vi "Get Output Values.vi"(8 "error in (no error)":errorcluster, 10 "Number of points":i32, 11 "Spectrum Recorder in":refnum<class "Spectrum Recorder.lvclass">) -> (0 "error out":errorcluster, 2 "Output values":dbl[](array[numeric]), 3 "Spectrum Recorder out":refnum<class "Spectrum Recorder.lvclass">)   [LabVIEW 2016, in "Spectrum Recorder.lvclass"]
uses:
  Spectrum Recorder.lvclass
  D:/github/Measure_core/Instrument Actor/Instrument Actor.lvclass
  Spectrum Recorder.lvclass/Spectrum Recorder.ctl
  Read Spectrum Recorder Configuration.vi
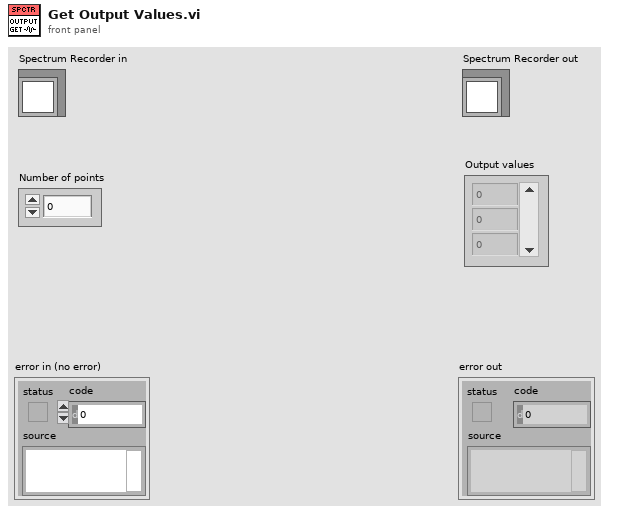
[diagram p1: front panel]
types:
  T1 = typedef "Spectrum Recorder Configuration.ctl" = cluster{"Start":dbl, "End":dbl, "Duration":dbl, "Filter time constant":dbl, "Repeat (-1: forever)":i32, "Update rate":dbl, "Data storage folder":path}
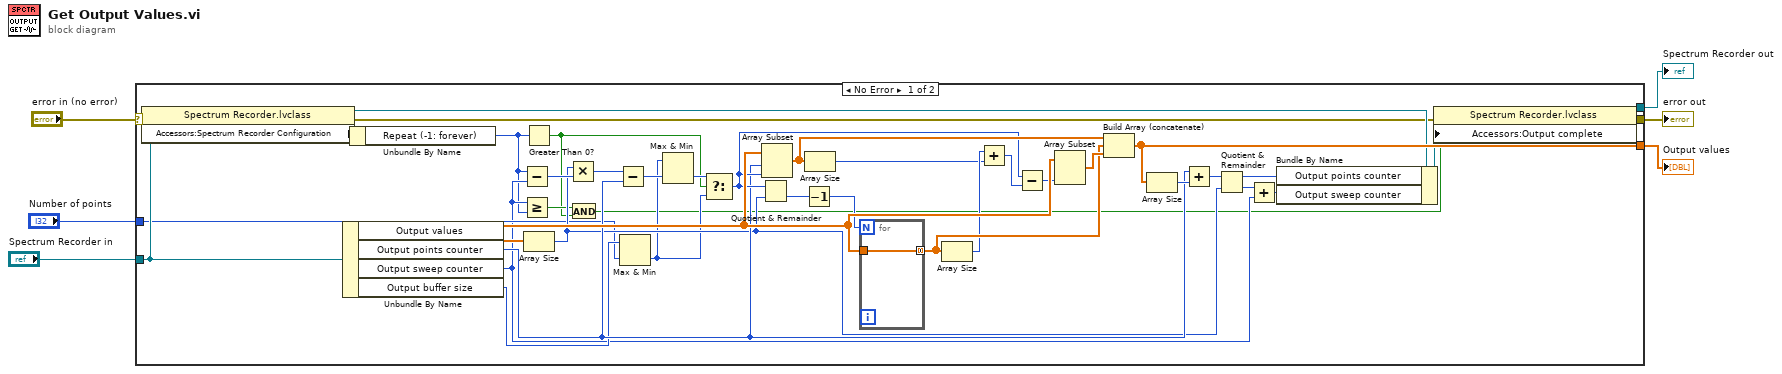
[diagram p0: block diagram]
diagram:
  n1 = case shown="No Error" "error in (no error)" {
    selector: "error in (no error)" -> [w14 w48]
    tunnel: [w10 w48] -> w5
    tunnel: [w8 w47] -> w3
    tunnel: "Spectrum Recorder in" -> [w45 w47]
    tunnel: "Number of points" -> [w20 _]
    tunnel: [w28 _] -> w1
    frame No Error {
      n2 = property class="Spectrum Recorder.lvclass"(reference=w45, error in=w14) -> (reference out=w15:refnum<class "Spectrum Recorder.lvclass">, error out=w13:errorcluster, "Accessors:Spectrum Recorder Configuration"=w12:T1)
      n3 = Unbundle By Name(w45) -> ("Output values"=w42:dbl[], "Output points counter"=w26:i32, "Output sweep counter"=w18:i32, "Output buffer size"=w21:i32)
      n4 = Unbundle By Name(w12) -> ("Repeat (-1: forever)"=w11:i32)
      n5 = Subtract(x=w11, y=w18) -> (x-y=w44:i32)
      n6 = Greater Or Equal?(x=w18, y=w11) -> (x >= y?=w17:bool)
      n7 = Greater Than 0?(x=w11) -> (x > 0?=w16:bool)
      n8 = Array Size(array=w42) -> (size(s)=w24:i32)
      n9 = Multiply(x=w24, y=w44) -> (x*y=w35:i32)
      n10 = And(x=w17, y=w16) -> (x .and. y?=w7:bool)
      n11 = Subtract(x=w35, y=w26) -> (x-y=w34:i32)
      n12 = Max & Min(x=w21, y=w20) -> (min(x,y)=w19:i32)  [unwired: 1 out]
      n13 = Max & Min(x=w19, y=w34) -> (min(x,y)=w32:i32)  [unwired: 1 out]
      n14 = Select(t=w32, s=w16, f=w19) -> (s? t:f=w31:i32)
      n15 = Quotient & Remainder(x=w31, y=w24) -> (floor(x/y)=w30:i32)  [unwired: 1 out]
      n16 = Array Subset(array=w42, index=w26, length=w31) -> (w40:dbl[])
      n17 = Decrement(x=w30) -> (x-1=w33:i32)
      n18 = Array Size(array=w40) -> (size(s)=w38:i32)
      n19 = for {
        N: w33 -> [_]
        tunnel: [w46] -> w41 mode=concatenating
        tunnel: w42 -> [w46]
      }
      n20 = Array Size(array=w41) -> (size(s)=w39:i32)
      n21 = Add(x=w39, y=w38) -> (x+y=w37:i32)
      n22 = Subtract(x=w31, y=w37) -> (x-y=w36:i32)
      n23 = Array Subset(array=w42, length=w36) -> (w43:dbl[])  [unwired: 1 in]
      n24 = Build Array (concatenate)(w40, w41, w43) -> (w28:dbl[])
      n25 = Array Size(array=w28) -> (size(s)=w27:i32)
      n26 = Add(x=w26, y=w27) -> (x+y=w25:i32)
      n27 = Quotient & Remainder(x=w25, y=w24) -> (x-y*floor(x/y)=w23:i32, floor(x/y)=w22:i32)
      n28 = Add(x=w22, y=w18) -> (x+y=w29:i32)
      n29 = Bundle By Name(cluster=w15, "Output points counter"=w23, "Output sweep counter"=w29) -> (w9:refnum<class "Spectrum Recorder.lvclass">)
      n30 = property class="Spectrum Recorder.lvclass"(reference=w9, error in=w13, "Accessors:Output complete"=w7) -> (reference out=w8:refnum<class "Spectrum Recorder.lvclass">, error out=w10:errorcluster)
    }
    frame Error {
    }
  }
  "error out" <- w5
  "Spectrum Recorder out" <- w3
  "Output values" <- w1
